vi "Factory.vi"() -> (3 "specific class reference":refnum<class "Camara.lvclass">)   [LabVIEW 2020]
uses:
  Clases/Abstracta/Camara/Camara.lvclass
panel:
  in  "Seleccionar":bool
  in  "Objeto a Instanciar":u16(ring) items=["FireWire.lvclass", "GigE.lvclass", "Simulada.lvclass", "Webcam.lvclass"]
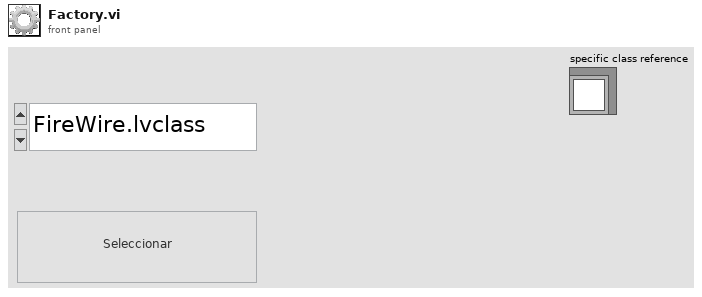
[diagram p1: front panel]
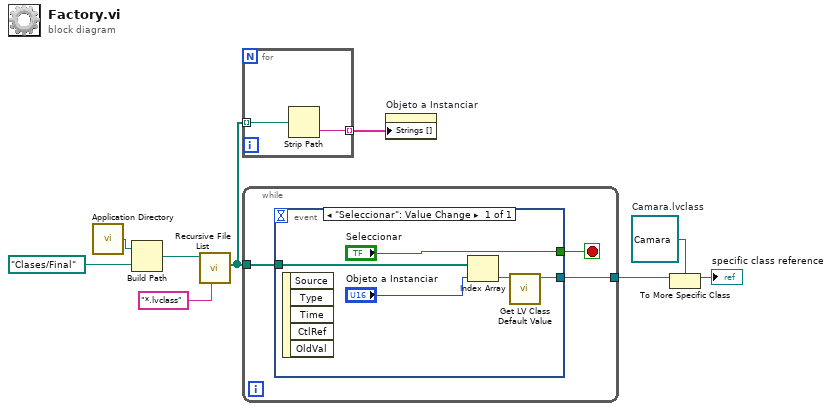
[diagram p0: block diagram]
diagram:
  w3 = refnum<class "Camara.lvclass"> refnum  # Camara.lvclass
  n1 = call <vilib>:"Application Directory.vi"() -> ("Application Directory"=w9:path)
  n2 = Build Path(base path=w9, name or relative path=path "Clases/Final") -> (appended path=w7:path)
  n3 = call <vilib>:"Recursive File List.vi"("pattern"="*.lvclass", "Folder Path"=w7) -> ("All Files in Dir"=w5:path[])  [unwired: 5 in, 4 out]
  n4 = for {
    tunnel: w5 -> [w11] mode=indexing
    tunnel: [w10] -> w6 mode=indexing
    n5 = Strip Path(path=w11) -> (name=w10:string)  [unwired: 1 out]
  }
  n6 = while {
    tunnel: w5 -> [w13]
    tunnel: [w12] -> w4
    stop <- w14 stop-if-true
    n7 = event shown="[0] \"Seleccionar\": Value Change" {
      selector: _ -> [_]
      dyn-events: _ -> [_]
      timeout: _ -> [_]
      tunnel: ["Seleccionar"] -> w14
      tunnel: w13 -> [w18]
      tunnel: [w15] -> w12
      event "Seleccionar": Value Change {
        n8 = event-data() -> ()  [unwired: 1 in, 5 out]
        n9 = Index Array(array=w18, index="Objeto a Instanciar") -> (element=w16:path)
        n10 = call <vilib>:"Get LV Class Default Value.vi"("class path"=w16) -> ("object"=w15:refnum<class>)  [unwired: 9 in, 1 out]
      }
    }
  }
  n11 = property on="Objeto a Instanciar" class="Ring (strict)"("Strings []"=w6) -> ()  [unwired: 2 in, 2 out]
  n12 = To More Specific Class(target class=w3, reference=w4) -> (specific class reference=→"specific class reference":refnum<class "Camara.lvclass">)  [unwired: 1 in, 1 out]
